vi "FanSpeedControl.vi"() -> ()   [LabVIEW 2020]
uses:
  C:/Users/Hannah/Documents/GitHub/pan-ASLM/LabVIEW camera PVCam/Dependencies/PVCamNET.dll
  Dependencies/PVCamNET.dll
panel:
  in  "?":bool
  out "Current Value":string
  in  "Fan Speed":string(combo)
  in  "?":bool
  # "FanSpeedControl.vi\n\nDescription:\nThis sample code lets the user control the fan speed. \n\nSteps to run:\n1. Click \"Run\"\n2. Click \"START\"\n3. Select Fan Speed\n4. Repeat step 2, observe changes in fan speed noise\n5. Click \"STOP\""
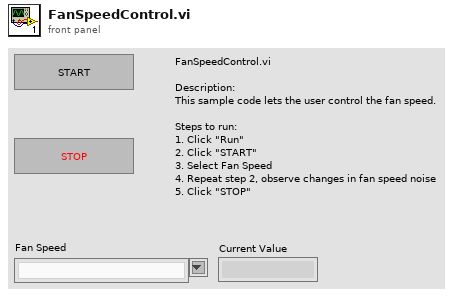
[diagram p1: front panel]
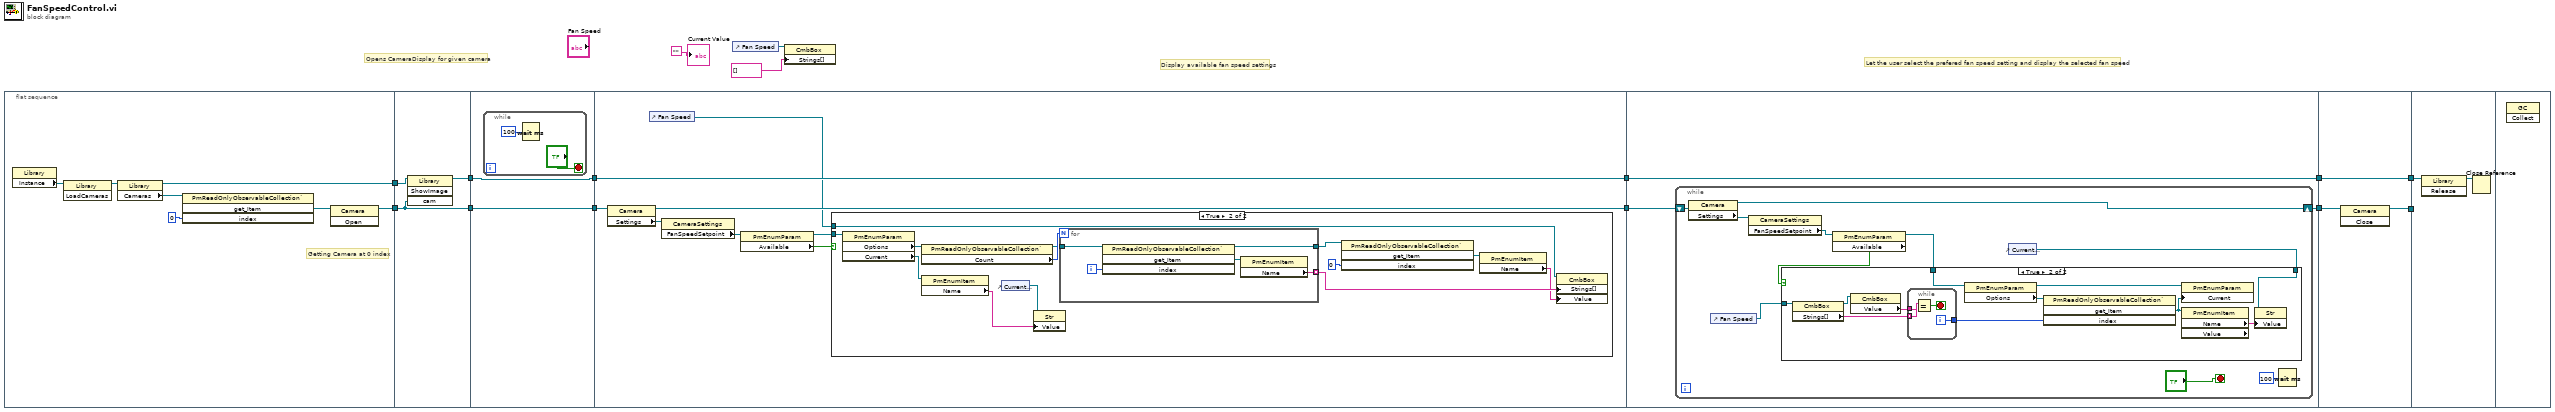
[diagram p0: block diagram]
diagram:
  # "Let the user select the prefered fan speed setting and display the selected fan speed"
  # "Display available fan speed settings"
  # "Opens CameraDisplay for given camera"
  n1 = flat-sequence {
    tunnel: [w18] -> w15
    tunnel: [w19] -> w14
    tunnel: w15 -> [w25]
    tunnel: w14 -> [w24]
    tunnel: [w24] -> w13
    tunnel: [w23] -> w12
    tunnel: w13 -> [w27]
    tunnel: [w27] -> w10
    tunnel: w12 -> [w26]
    tunnel: [w26] -> w11
    tunnel: [w37] -> w7
    tunnel: [w36] -> w5
    tunnel: w11 -> [w36]
    tunnel: w10 -> [w35]
    tunnel: w7 -> [w58]
    tunnel: [w56] -> w6
    tunnel: w5 -> [w57]
    tunnel: [w57] -> w4
    tunnel: [w85] -> w9
    tunnel: [w84] -> w8
    tunnel: w4 -> [w84]
    tunnel: w6 -> [w86]
    tunnel: w9 -> [_]
    tunnel: w8 -> [w88]
    frame #0 {
      # "Getting Camera at 0 index"
      n2 = property class="Library"() -> ("Instance"=w17:refnum<k24>)  [unwired: 2 in, 2 out]
      n3 = invoke class="Library" method="LoadCameras"(reference=w17) -> (reference out=w16:refnum<k24>)  [unwired: 2 in, 2 out]
      n4 = property class="Library"(reference=w16) -> (reference out=w18:refnum<k24>, "Cameras"=w22:refnum<k24>)  [unwired: 1 in, 1 out]
      n5 = invoke class="PmReadOnlyObservableCollection`" method="get_Item"(reference=w22, "index"=0) -> ("get_Item"=w20:refnum<k24>)  [unwired: 2 in, 3 out]
      n6 = invoke class="Camera" method="Open"(reference=w20) -> (reference out=w19:refnum<k24>)  [unwired: 2 in, 2 out]
    }
    frame #1 {
      n7 = invoke class="Library" method="ShowImage"(reference=w25, "cam"=w24) -> (reference out=w23:refnum<k24>)  [unwired: 2 in, 3 out]
    }
    frame #2 {
      n8 = while {
        stop <- "?" stop-if-true
        n9 = Wait (ms)(milliseconds to wait=u32 100) -> ()  [unwired: 1 out]
      }
    }
    frame #3 {
      n10 = property class="Camera"(reference=w35) -> (reference out=w37:refnum<k24>, "Settings"=w34:refnum<k24>)  [unwired: 1 in, 1 out]
      n11 = control-ref of="Fan Speed"() -> (w30:refnum<vi>)
      n12 = property class="CameraSettings"(reference=w34) -> ("FanSpeedSetpoint"=w33:refnum<k24>)  [unwired: 1 in, 2 out]
      n13 = property class="PmEnumParam"(reference=w33) -> (reference out=w31:refnum<k24>, "Available"=w32:bool)  [unwired: 1 in, 1 out]
      n14 = case shown="True" w32 {
        tunnel: w30 -> [_ w42]
        tunnel: w31 -> [_ w41]
        frame False {
        }
        frame True {
          n15 = property class="PmEnumParam"(reference=w41) -> ("Options"=w50:refnum<k24>, "Current"=w40:refnum<k24>)  [unwired: 1 in, 2 out]
          n16 = property class="PmReadOnlyObservableCollection`"(reference=w50) -> (reference out=w48:refnum<k24>, "Count"=w49:i32)  [unwired: 1 in, 1 out]
          n17 = property class="PmEnumItem"(reference=w40) -> ("Name"=w38:string)  [unwired: 1 in, 2 out]
          n18 = control-ref of="Current Value"() -> (w39:refnum<vi>)
          n19 = property class="Str"(reference=w39, "Value"=w38) -> ()  [unwired: 1 in, 2 out]
          n20 = for {
            N: w49 -> [_]
            tunnel: w48 -> [w55]
            tunnel: [w52] -> w46
            tunnel: [w51] -> w47 mode=indexing
            i -> [w54]
            n21 = invoke class="PmReadOnlyObservableCollection`" method="get_Item"(reference=w55, "index"=w54) -> (reference out=w52:refnum<k24>, "get_Item"=w53:refnum<k24>)  [unwired: 2 in, 2 out]
            n22 = property class="PmEnumItem"(reference=w53) -> ("Name"=w51:string)  [unwired: 1 in, 2 out]
          }
          n23 = invoke class="PmReadOnlyObservableCollection`" method="get_Item"(reference=w46, "index"=0) -> ("get_Item"=w44:refnum<k24>)  [unwired: 2 in, 3 out]
          n24 = property class="PmEnumItem"(reference=w44) -> ("Name"=w43:string)  [unwired: 1 in, 2 out]
          n25 = property class="CmbBox"(reference=w42, "Strings[]"=w47, "Value"=w43) -> ()  [unwired: 1 in, 2 out]
        }
      }
    }
    frame #4 {
      n26 = while {
        shift-right: [w61] -> w56
        shift-left: w58 -> [w67]
        stop <- "?" stop-if-true
        n27 = property class="Camera"(reference=w67) -> (reference out=w61:refnum<k24>, "Settings"=w68:refnum<k24>)  [unwired: 1 in, 1 out]
        n28 = control-ref of="Fan Speed"() -> (w63:refnum<vi>)
        n29 = property class="CameraSettings"(reference=w68) -> ("FanSpeedSetpoint"=w66:refnum<k24>)  [unwired: 1 in, 2 out]
        n30 = property class="PmEnumParam"(reference=w66) -> (reference out=w64:refnum<k24>, "Available"=w65:bool)  [unwired: 1 in, 1 out]
        n31 = control-ref of="Current Value"() -> (w62:refnum<vi>)
        n32 = case shown="True" w65 {
          tunnel: w64 -> [_ w78]
          tunnel: w63 -> [_ w74]
          tunnel: w62 -> [_ w71]
          frame False {
          }
          frame True {
            n33 = property class="CmbBox"(reference=w74) -> (reference out=w73:refnum<vi>, "Strings[]"=w79:string[])  [unwired: 1 in, 1 out]
            n34 = property class="CmbBox"(reference=w73) -> ("Value"=w72:string)  [unwired: 1 in, 2 out]
            n35 = while {
              tunnel: w79 -> [w83] mode=indexing
              tunnel: [w81] -> w76
              tunnel: w72 -> [w80]
              i -> [w81]
              stop <- w82 stop-if-true
              n36 = Equal?(x=w83, y=w80) -> (x = y?=w82:bool)
            }
            n37 = property class="PmEnumParam"(reference=w78) -> (reference out=w75:refnum<k24>, "Options"=w77:refnum<k24>)  [unwired: 1 in, 1 out]
            n38 = invoke class="PmReadOnlyObservableCollection`" method="get_Item"(reference=w77, "index"=w76) -> ("get_Item"=w69:refnum<k24>)  [unwired: 2 in, 3 out]
            n39 = property class="PmEnumParam"(reference=w75, "Current"=w69) -> ()  [unwired: 1 in, 2 out]
            n40 = property class="PmEnumItem" props=["Name", "Value"](reference=w69) -> ("Name"=w70:string)  [unwired: 1 in, 3 out]
            n41 = property class="Str"(reference=w71, "Value"=w70) -> ()  [unwired: 1 in, 2 out]
          }
        }
        n42 = Wait (ms)(milliseconds to wait=u32 100) -> ()  [unwired: 1 out]
      }
    }
    frame #5 {
      n43 = invoke class="Camera" method="Close"(reference=w86) -> (reference out=w85:refnum<k24>)  [unwired: 2 in, 2 out]
    }
    frame #6 {
      n44 = invoke class="Library" method="Release"(reference=w88) -> (reference out=w87:refnum<k24>)  [unwired: 2 in, 2 out]
      n45 = Close Reference(reference=w87) -> ()  [unwired: 1 in, 1 out]
    }
    frame #7 {
      n46 = invoke class="GC" method="Collect"() -> ()  [unwired: 3 in, 3 out]
    }
  }
  n47 = control-ref of="Fan Speed"() -> (w2:refnum<vi>)
  n48 = property class="CmbBox"(reference=w2, "Strings[]"=string[] [] ("Strings []")) -> ()  [unwired: 1 in, 2 out]
  "Current Value" <- ""
